vi "Dashboard Main.vi"() -> ()   [LabVIEW 2012]
uses:
  <vilib>/event_ctls.llb/eventvkey.ctl
  <vilib>/Utility/config.llb/Read Key (String).vi
  <vilib>/Utility/config.llb/Read Key (I32).vi
  <vilib>/Utility/config.llb/Write Key (String).vi
  <vilib>/Utility/config.llb/Write Key (I32).vi
  <vilib>/Utility/config.llb/NI_LVConfig.lvlib
panel:
  in  "Camera Settings":T1={"Frate Rate"=30, "Compression"=30, "Size"=1} {"Frate Rate" scale=1.0..30.0; "Size" items=["640x480", "320x240", "160x120"]}
  out "Mode":T2(ring)=enum."Auto Disabled"
  out "Camera IP":string
  in  "Dashboard Tab":T3(tab)
  in  "Reverse":bool
  in  "Control Mode":string(combo)="Tank: Dual Joystick"
  out "Lifting?":bool
  out "Lifting Enabled?":bool caption="Launching Enabled"
  out "Ready to fire?":bool
  out "Firing?":bool
  out "Launching Enabled?":bool caption="Launching Enabled"
  out "JS1 Z":dbl(slide) scale=-1.0..1.0 scale format="%#_2e"
  out "JS2 Z":dbl(slide) scale=-1.0..1.0 scale format="%#_2e"
  out "Joystick 1":cluster{"X":dbl, "Y":dbl}[](graph)
  out "Joystick 2":cluster{"X":dbl, "Y":dbl}[](graph)
  out "JS Buttons 1":T4
  out "JS Buttons 2":T4
  out "MotorSlide4":dbl(slide) scale=-1.0..1.0 scale format="%#_2e"
  out "MotorSlide3":dbl(slide) scale=-1.0..1.0 scale format="%#_2e"
  out "MotorSlide2":dbl(slide) scale=-1.0..1.0 scale format="%#_2e"
  in  "MotorName3":string="Front Left"
  in  "MotorName4":string="Front Right"
  in  "MotorName1":string="Rear Left"
  in  "MotorName2":string="Rear Right"
  out "MotorChart4":dbl(graph)
  out "MotorChart3":dbl(graph)
  out "MotorChart2":dbl(graph)
  out "MotorSlide1":dbl(slide) scale=-1.0..1.0 scale format="%#_2e"
  out "MotorChart1":dbl(graph)
  out "Battery Value":dbl(slide) scale=0.0..14.0 scale format="%#_2e"
  out "Battery":sgl(graph)
  out "Robot IP":string
  out "Motor Speed":dbl
  out "Throttle Speed":dbl
  in  "DB Camera Config":bool
  in  "Enable":bool=TRUE
  out "Mbps 2":dbl format="%#.1g"
  out "fps":dbl format="%#.1g"
  out "Mbps":bool
  in  "Slider":dbl(slide) scale=0.0..100.0 scale format="%#_3g"
  in  "On/Off":bool caption="Solenoid"
  in  "Test Name":u16(ring) items=["Select the test to run...", "Example Test", "-------------------------------", "List of tests is built in robot code.", "Replace with your own automated tests."]
  in  "Test Tree":string(tree)
  in  "Motor":cluster{"Value":dbl, "Enable":bool} {"Value" scale=-1.0..1.0 scale format="%#_3g"}
  out "Progress":T5 {"Test Progress" scale=0.0..100.0}
  in  "Rev/Fwd":cluster{"Forward":bool, "Reverse":bool}
  in  "Ring":u16(ring) items=["Auto", "Fixed indoor", "Fixed outdoor 1", "Fixed outdoor 2", "Fixed fluorescent 1", "Fixed fluorescent 2", "Hold current"]
  in  "Listbox":i32(listbox)
  in  "Viewer":T6(tab)
  out "Image Error Message":string="Timeout in Camera Communications"
  out "Camera Image":T7(plugin-control)
  out "Buttons 1":cluster{"1":bool, "2":bool, "3":bool}
  out "Kinect 1":cluster{"X":dbl, "Y":dbl, "Z":dbl} {"X" scale=1.0..-1.0; "Y" scale=1.0..-1.0; "Z" scale=1.0..-1.0}
  out "Buttons 2":cluster{"1":bool, "2":bool, "3":bool}
  out "Kinect 2":cluster{"X":dbl, "Y":dbl, "Z":dbl} {"X" scale=1.0..-1.0; "Y" scale=1.0..-1.0; "Z" scale=1.0..-1.0}
  out "Version":string
  out "Skeleton Picture":picture
  out "Players":i8
  out "Tree":string(tree)
  # "Robot IP:"
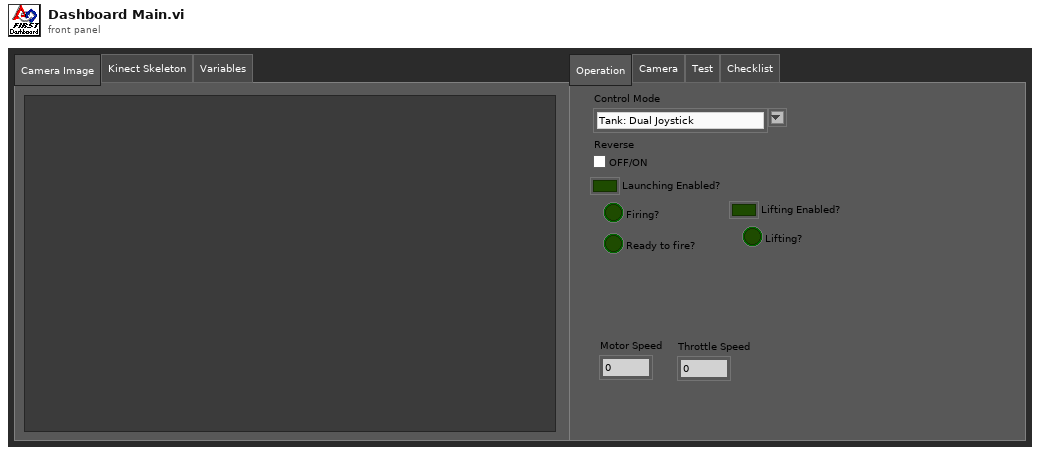
[diagram p1: front panel]
types:
  T1 = cluster{"Frate Rate":i32, "Compression":i32, "Size":u16}
  T2 = enum8{"Tele-Op Disabled", "Tele-Op Enabled", "Auto Disabled", "Auto Enabled", "Test Disabled", "Test Enabled", ""}
  T3 = enum32{"Operation", "Camera", "Test", "Checklist"}
  T4 = cluster{bool, bool, bool, bool, bool, bool, bool, bool, bool, bool, bool, bool}
  T5 = cluster{"Test Progress":u8, "Test Progress Text":string}
  T6 = enum32{"Camera Image", "Kinect Skeleton", "Variables"}
  T7 = typedef "IMAQ Image.ctl" = refnum<image>
  T8 = typedef "Image Type" = u32
  T9 = typedef "LVBoundsTypeDef.ctl" = cluster{"Width":u32, "Height":u32}
  T10 = typedef "SkeletonTrackState.ctl" = enum32{"NotTracked", "PositionOnly", "Tracked"}
  T11 = cluster{"TrackingState":u8[], "Position":cluster{"x":sgl, "y":sgl, "z":sgl}, cluster{"x":sgl, "y":sgl, "z":sgl, sgl}[], "TrackState":T10}
  T12 = cluster{cluster{"ScaledToPercentRange":dbl, "ScaledToPercentRange":dbl, "ScaledToPercentRange":dbl}, cluster{bool, bool, bool}}[]
  T13 = cluster{cluster{"ScaledToPercentRange":dbl, "ScaledToPercentRange":dbl, "ScaledToPercentRange":dbl}, cluster{bool, bool, bool}}
  T14 = cluster{"ScaledToPercentRange":dbl, "ScaledToPercentRange":dbl, "ScaledToPercentRange":dbl}
  T15 = typedef "LVRectTypeDef.ctl" = cluster{"Left":i16, "Top":i16, "Right":i16, "Bottom":i16}
  T16 = cluster{"Competition mode":bool, "Robot Link":bool, "Autonomous":bool, "Enabled":bool, "E-Stop":bool, "Simulated":bool, "TestMode":bool, "Docked Window":bool}
  T17 = cluster{"Boolean Array[0]":bool, "Boolean Array[1]":bool, "Boolean Array[2]":bool, "Boolean Array[3]":bool, "Boolean Array[4]":bool, "Boolean Array[5]":bool, "Boolean Array[6]":bool, "Boolean Array[7]":bool, "Boolean Array[8]":bool, "Boolean Array[9]":bool, "Boolean Array[10]":bool, "Boolean Array[11]":bool}
  T18 = typedef "NI_LVConfig.lvlib/Config Data RefNum.ctl" = refnum<k1>
  T19 = typedef "eventvkey.ctl" = enum16{"ASCII", "Enter", "Return", "Shift", "Ctrl", "Alt", "Cmd", "Opt", "Caps", "NumLock", "Clear", "Break", "Up", "Down", "Left", "Right", "Insert", "Delete", "Home", "End", "PageUp", "PageDown", "Escape", "Help", "Pause", "ScrollLock", "F1", "F2", "F3", "F4", "F5", "F6", "F7", "F8", "F9", "F10", "F11", "F12", "F13", "F14", "F15", "F16", "F17", "F18", "F19", "F20", "F21", "F22", "F23", "F24", "Play", "VolumeUp", "VolumeDown", "Mute", "Two Byte Char"}
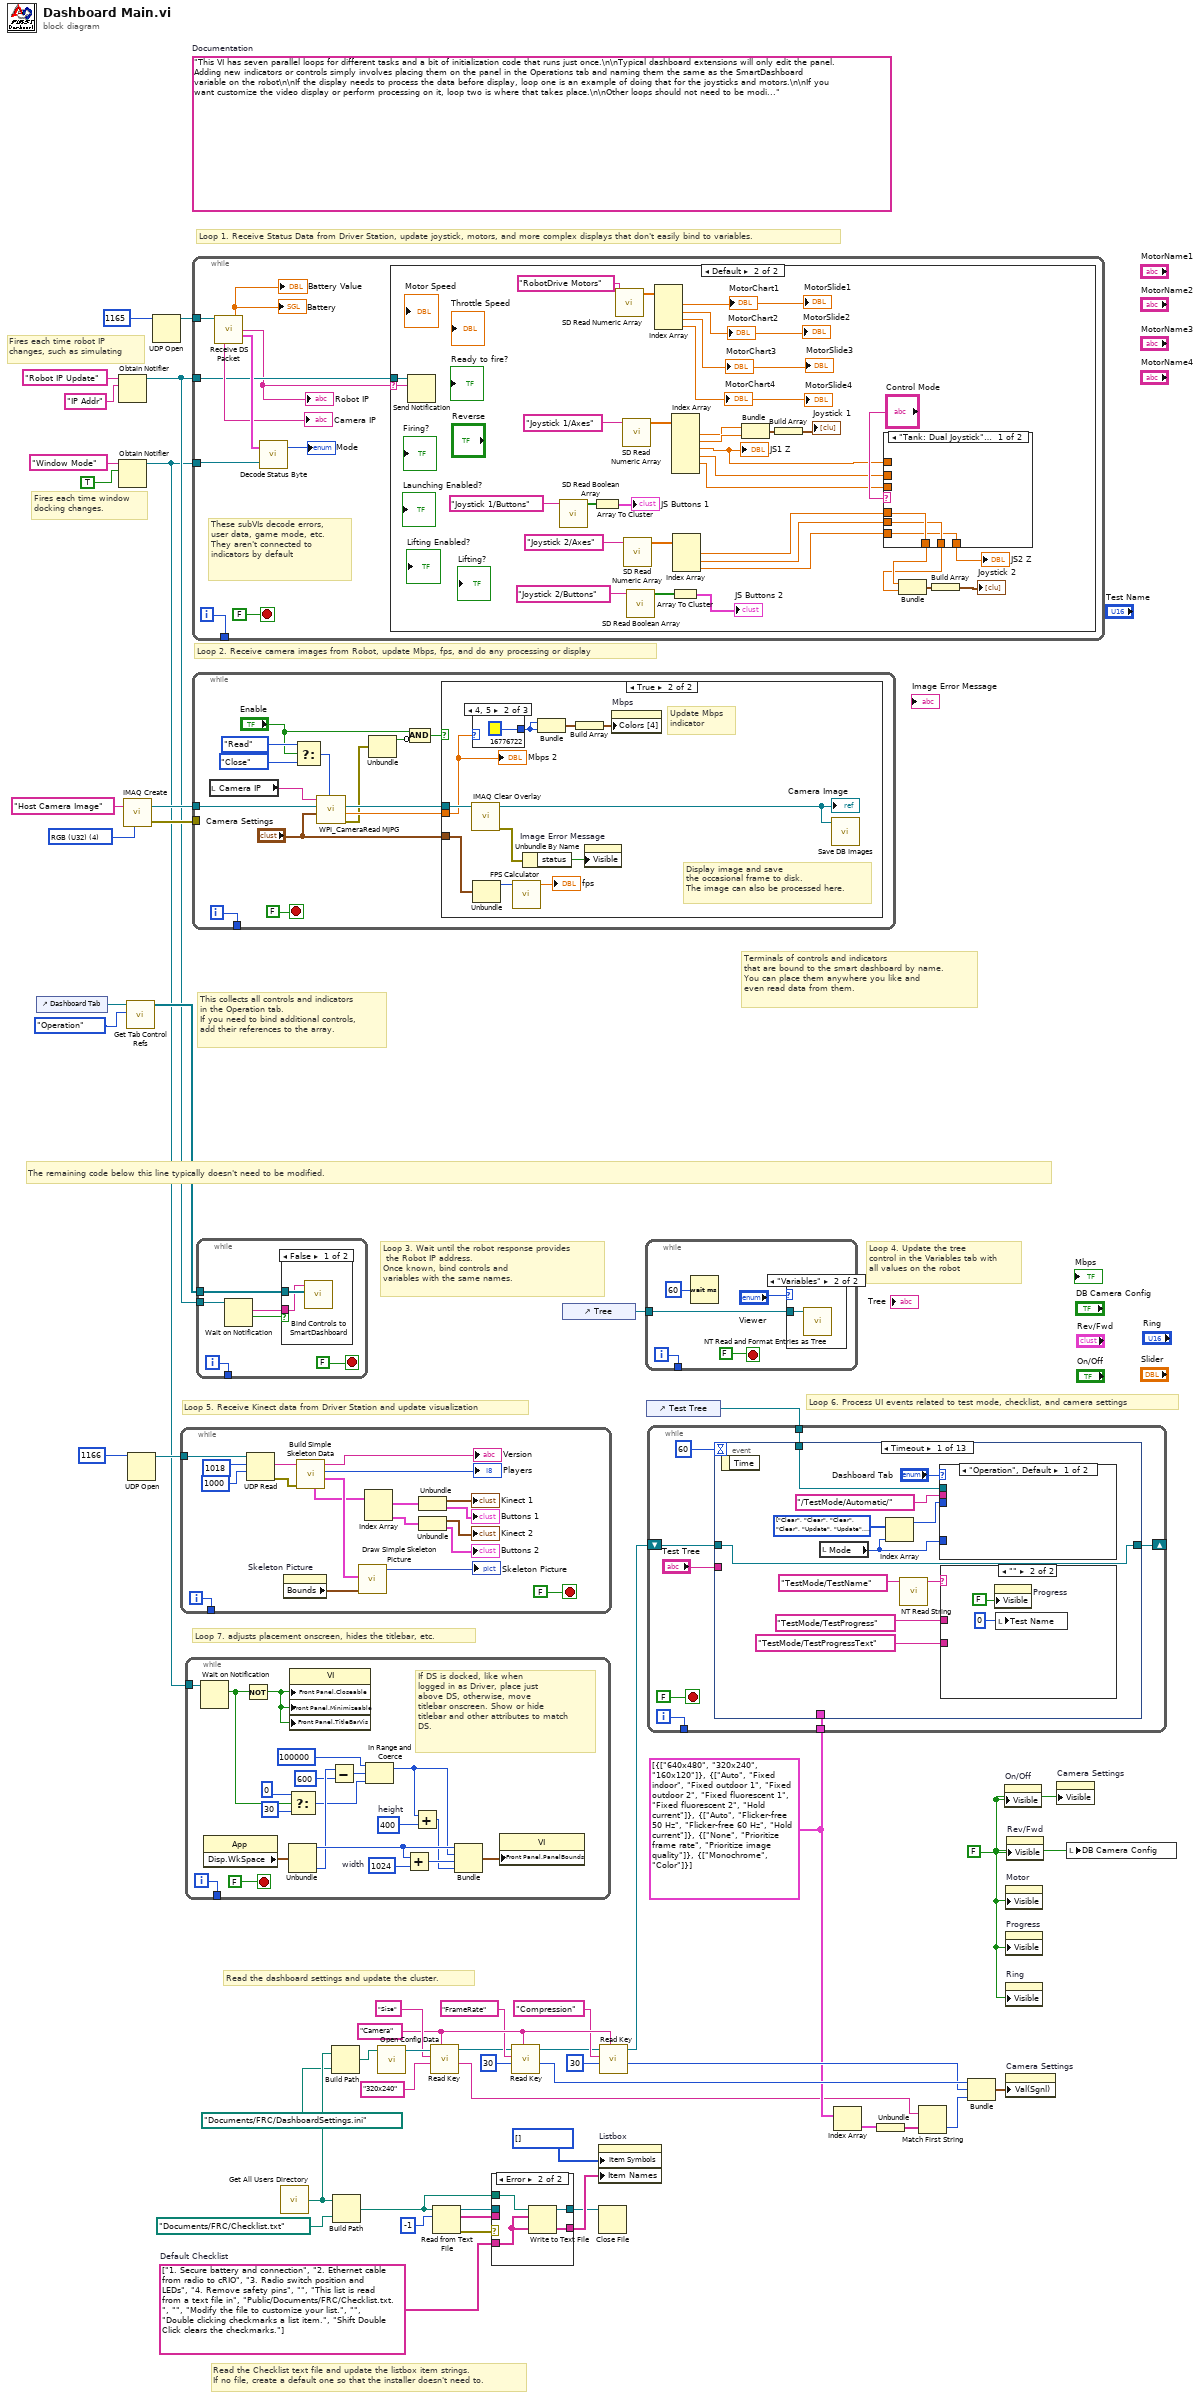
[diagram p0: block diagram]
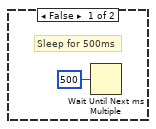
[diagram p3: hidden frame]
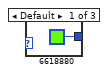
[diagram p4: hidden frame]
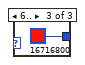
[diagram p5: hidden frame]
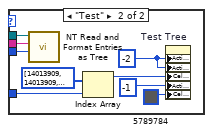
[diagram p7: hidden frame]
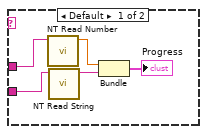
[diagram p8: hidden frame]
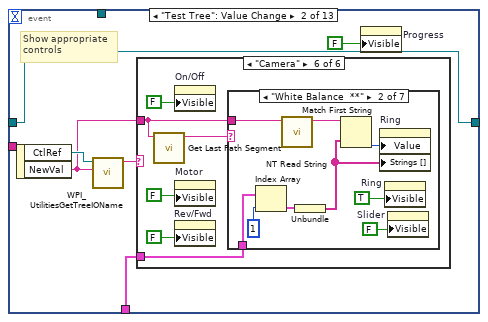
[diagram p9: hidden frame]
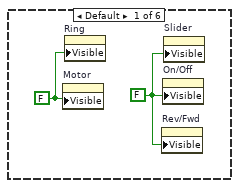
[diagram p10: hidden frame]
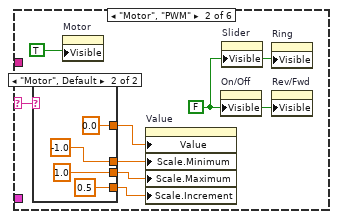
[diagram p11: hidden frame]
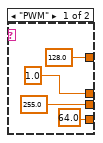
[diagram p12: hidden frame]
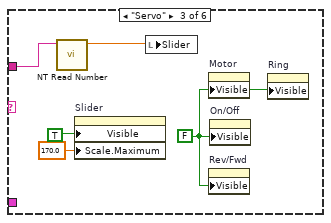
[diagram p13: hidden frame]
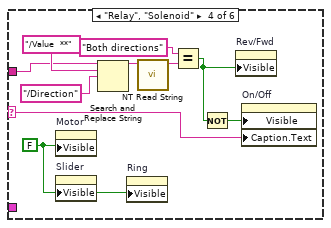
[diagram p14: hidden frame]
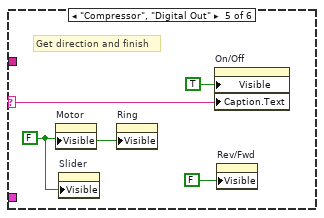
[diagram p15: hidden frame]
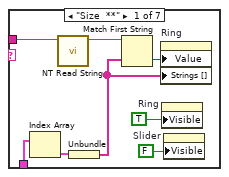
[diagram p16: hidden frame]
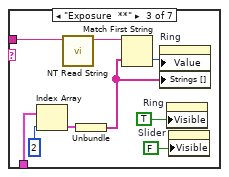
[diagram p17: hidden frame]
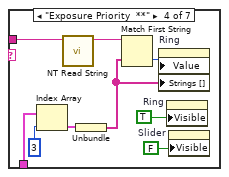
[diagram p18: hidden frame]
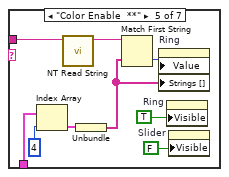
[diagram p19: hidden frame]
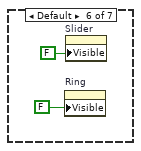
[diagram p20: hidden frame]
diagram:
  w21 = "Camera"
  w13 = cluster{string[]}[] [{["640x480", "320x240", "160x120"]}, {["Auto", "Fixed indoor", "Fixed outdoor 1", "Fixed outdoor 2", "Fixed fluorescent 1", "Fixed fluorescent 2", "Hold current"]}, {["Auto", "Flicker-free 50 Hz", "Flicker-free 60 Hz", "Hold current"]}, {["None", "Prioritize frame rate", "Prioritize image quality"]}, {["Monochrome", "Color"]}]
  w29 = string[] ["1. Secure battery and connection", "2. Ethernet cable from radio to cRIO", "3. Radio switch position and LEDs", "4. Remove safety pins", "", "This list is read from a text file in", "Public/Documents/FRC/Checklist.txt.", "", "Modify the file to customize your list.", "", "Double clicking checkmarks a list item.", "Shift Double Click clears the checkmarks."]  # Default Checklist
  w27 = FALSE ("Visible")
  (unwired) "This VI has seven parallel loops for different tasks and a bit of initialization code that runs just once.\n\nTypical dashboard extensions will only edit the panel. Adding new indicators or controls simply involves placing them on the panel in the Operations tab and naming them the same as the SmartDashboard variable on the robot\n\nIf the display needs to process the data before display, loop one is an example of doing that for the joysticks and motors.\n\nIf you want customize the video display or perform processing on it, loop two is where that takes place.\n\nOther loops should not need to be modified. They are pretty standard, and document the task they perform."  # Documentation
  w50 = T8 4 items=["Grayscale (U8)", "Grayscale (I16)", "Grayscale (SGL)", "Complex (CSG)", "RGB (U32)", "HSL (U32)", "RGB (U64)"] ("Image Type")
  # "Fires each time robot IP\nchanges, such as simulating"
  # "Fires each time window\ndocking changes."
  # "Read the Checklist text file and update the listbox item strings.\nIf no file, create a default one so that the installer doesn't need to."
  # "This collects all controls and indicators\nin the Operation tab.\nIf you need to bind additional controls,\nadd their references to the array."
  # "The remaining code below this line typically doesn't need to be modified."
  # "Loop 6. Process UI events related to test mode, checklist, and camera settings"
  # "Read the dashboard settings and update the cluster."
  # "Terminals of controls and indicators\nthat are bound to the smart dashboard by name.\nYou can place them anywhere you like and\neven read data from them."
  # "Loop 4. Update the tree\ncontrol in the Variables tab with\nall values on the robot"
  # "Loop 3. Wait until the robot response provides\n the Robot IP address.\nOnce known, bind controls and\nvariables with the same names."
  # "Loop 5. Receive Kinect data from Driver Station and update visualization"
  # "Loop 7. adjusts placement onscreen, hides the titlebar, etc."
  # "Loop 1. Receive Status Data from Driver Station, update joystick, motors, and more complex displays that don't easily bind to variables."
  # "Loop 2. Receive camera images from Robot, update Mbps, fps, and do any processing or display"
  n1 = control-ref of="Dashboard Tab"() -> (w43:refnum<vi>)
  n2 = Obtain Notifier(name (unnamed)="Robot IP Update", notification data type="IP Addr" ("name (unnamed)")) -> (notifier out=w40:refnum<notifier>)  [unwired: 2 in, 2 out]
  n3 = Obtain Notifier(name (unnamed)="Window Mode", notification data type=TRUE) -> (notifier out=w33:refnum<notifier>)  [unwired: 2 in, 2 out]
  n4 = call "IMAQ Create"("Image Name"="Host Camera Image", "Image Type"=w50) -> ("New Image"=w48:T7, "error out"=w47:errorcluster)  [unwired: 2 in, 1 out]
  n5 = call <vilib>:"Get Tab Control Refs.vi"("Page Index"=enum32{"Operation", "Test"}."Operation" ("Dashboard Tab"), "TabControl in"=w43) -> ("ControlsOnPage"=w44:refnum<vi>[])  [unwired: 9 in]
  n6 = UDP Open(11:u16 1166 ("port")) -> (port=w45:refnum<k16>)  [unwired: 2 in, 4 out]
  n7 = UDP Open(11:u16 1165 ("port")) -> (port=w51:refnum<k16>)  [unwired: 2 in, 4 out]
  n8 = while {
    tunnel: w45 -> [w69]
    tunnel: [w54] -> _
    i -> [w54]
    stop <- FALSE stop-if-true
    n9 = UDP Read(connection ID=w69, max size (548)=1018 ("bytes to read"), timeout ms (25000)=1000) -> (data out=w63:string, error out=w53:errorcluster)  [unwired: 1 in, 3 out]
    n10 = property on="Skeleton Picture" class="Pict"() -> ("Bounds"=w65:T9)  [unwired: 2 in, 2 out]
    n11 = call "Build Simple Skeleton Data.vi"("error in (no error)"=w53, "data in"=w63) -> ("Skeleton Data"=w64:T11, "NumPlayers"=→"Players":i8, "Version String"=→"Version":string, "Simple Joystick Info"=w61:T12)  [unwired: 5 in, 1 out]
    n12 = call "Draw Simple Skeleton Picture.vi"("Bounds"=w65, "Simple Skeleton"=w64) -> ("new picture out"=→"Skeleton Picture":picture)  [unwired: 9 in]
    n13 = Index Array(array=w61) -> (element #1=w60:T13, element #2=w59:T13)  [unwired: 2 in]
    n14 = Unbundle(w60) -> (→"Kinect 1":T14, →"Buttons 1":cluster{bool, bool, bool})
    n15 = Unbundle(w59) -> (→"Kinect 2":T14, →"Buttons 2":cluster{bool, bool, bool})
  }
  n16 = while {
    tunnel: w33 -> [w90]
    tunnel: [w88] -> _
    i -> [w88]
    stop <- FALSE stop-if-true
    w80 = 1024  # width
    w83 = 400  # height
    # "If DS is docked, like when\nlogged in as Driver, place just\nabove DS, otherwise, move\ntitlebar onscreen. Show or hide\ntitlebar and other attributes to match\nDS."
    n17 = Wait on Notification(notifier=w90) -> (notification=w75:bool)  [unwired: 3 in, 3 out]
    n18 = property class="App"() -> ("Disp.WkSpace"=w86:T15)  [unwired: 2 in, 2 out]
    n19 = Not(x=w75) -> (.not. x?=w89:bool)
    n20 = Unbundle(w86) -> ("Left"=w84:i16, "Bottom"=w81:i16)  [unwired: 2 out]
    n21 = Select(t=0, s=w75, f=30) -> (s? t:f=w74:i32)
    n22 = property class="VI"("Front Panel.Closeable"=w89, "Front Panel.Minimizeable"=w89, "Front Panel.TitleBarVis"=w89) -> ()  [unwired: 2 in, 2 out]
    n23 = Subtract(x=w81, y=600) -> (x-y=w78:i32)
    n24 = In Range and Coerce(upper limit=100000, x=w78, lower limit=w74) -> (coerced(x)=w72:i32)  [unwired: 1 out]
    n25 = Add(x=w84, y=w80) -> (x+y=w85:i32)
    n26 = Add(x=w72, y=w83) -> (x+y=w82:i32)
    n27 = Bundle("Left"=w84, w72, w85, w82) -> (w87:cluster{"Left":i16, i32, i32, i32})  [unwired: 1 out]
    n28 = property class="VI"("Front Panel.PanelBounds"=w87) -> ()  [unwired: 2 in, 2 out]
  }
  n29 = while {
    tunnel: w48 -> [w101]
    tunnel: w47 -> [_]
    tunnel: [w104] -> _
    i -> [w104]
    stop <- FALSE stop-if-true
    n30 = local read "Camera IP"() -> (w103:string)
    n31 = Select(t=enum16{"Read", "Reopen", "Close"}."Read" ("Operation"), s="Enable", f=enum16{"Read", "Reopen", "Close"}."Close" ("Operation")) -> (s? t:f=w96:enum16{"Read", "Reopen", "Close"})
    n32 = call <vilib>:"WPI_CameraRead MJPG.vi"("Operation"=w96, "Camera Settings"="Camera Settings", "Image"=w101, "address"=w103) -> ("error out"=w95:errorcluster, "Bandwidth (kbps)"=w99:dbl, "Image Out"=w100:T7)  [unwired: 5 in]
    n33 = Unbundle(w95) -> ("status"=w93:bool)  [unwired: 2 out]
    n34 = Compound Arithmetic op=AND("Enable", invert w93) -> (w92:bool)
    n35 = case shown="True" w92 {
      tunnel: "Camera Settings" -> [_ w108]
      tunnel: w100 -> [_ w111]
      tunnel: w99 -> [_ w110]
      frame False {
        # "Sleep for 500ms"
        n36 = Wait Until Next ms Multiple(millisecond multiple=u32 500) -> ()  [unwired: 1 out]
      }
      frame True {
        # "Display image and save\nthe occasional frame to disk.\nThe image can also be processed here."
        # "Update Mbps\nindicator"
        n37 = call "IMAQ Clear Overlay"("Image"=w111) -> ("error out"=w116:errorcluster, "Image Out"=w115:T7)  [unwired: 2 in, 7 out]
        "Camera Image" <- w115
        n38 = case shown="4, 5" w110 {
          tunnel: [u32 6618880 ("Color Box") u32 16776722 ("Color Box") u32 16716800 ("Color Box")] -> w112
          frame Default {
          }
          frame 4, 5 {
          }
          frame 6.. {
          }
        }
        n39 = Unbundle(w108) -> ("Frate Rate"=w107:i32)  [unwired: 2 out]
        n40 = call "FPS Calculator.vi"("Average Count"=w107) -> ("fps"=→"fps":dbl)  [unwired: 10 in]
        n41 = Unbundle By Name(w116) -> ("status"=w117:bool)
        n42 = Bundle("Color Box"=w112, "Color Box"=w112) -> (w114:cluster{"Color Box":u32, "Color Box":u32})  [unwired: 1 out]
        n43 = Build Array(w114) -> (w113:cluster{"Color Box":u32, "Color Box":u32}[])
        n44 = property on="Image Error Message" class="Str"("Visible"=w117) -> ()  [unwired: 2 in, 2 out]
        n45 = property on="Mbps" class="Bool (strict)"("Colors [4]"=w113) -> ()  [unwired: 2 in, 2 out]
        n46 = call "Save DB Images.vi"("Image"=w115) -> ()  [unwired: 2 in, 1 out]
        "Mbps 2" <- w110
      }
    }
  }
  n47 = while {
    tunnel: w51 -> [w128]
    tunnel: w40 -> [w122]
    tunnel: w33 -> [w126]
    tunnel: [w123] -> _
    i -> [w123]
    stop <- FALSE stop-if-true
    # "These subVIs decode errors, user data, game mode, etc.\nThey aren't connected to indicators by default"
    n48 = call "Receive DS Packet.vi"("Recv Socket"=w128) -> ("Battery"=→"Battery" →"Battery Value":sgl, "Robot IP Address"=w121:string, "Status"=w129:T16, "Camera IP Address"=→"Camera IP":string)  [unwired: 1 in, 10 out]
    "Robot IP" <- w121
    n49 = call "Decode Status Byte.vi"("Window Mode Notifier"=w126, "Status"=w129) -> ("Mode"=→"Mode":T2)  [unwired: 1 out]
    n50 = case shown="Default" w121 {
      selector: w121 -> [_ w142]
      tunnel: w122 -> [_ w143]
      frame "0.0.0.0" {
        # "Robot not responding, don't poll the variables"
      }
      frame Default {
        n51 = Send Notification(notification=w142, notifier=w143) -> ()  [unwired: 1 in, 2 out]
        n52 = call <vilib>:"SD Read Boolean Array.vi"("Name"="Joystick 1/Buttons") -> ("Boolean Array"=w156:bool[])  [unwired: 8 in, 2 out]
        n53 = Array To Cluster(array=w156) -> (cluster=→"JS Buttons 1":T17)
        n54 = call <vilib>:"SD Read Numeric Array.vi"("Name"="RobotDrive Motors") -> ("Numeric Array"=w161:dbl[])  [unwired: 8 in, 2 out]
        n55 = call <vilib>:"SD Read Numeric Array.vi"("Name"="Joystick 1/Axes") -> ("Numeric Array"=w154:dbl[])  [unwired: 8 in, 2 out]
        n56 = call <vilib>:"SD Read Numeric Array.vi"("Name"="Joystick 2/Axes") -> ("Numeric Array"=w149:dbl[])  [unwired: 8 in, 2 out]
        n57 = call <vilib>:"SD Read Boolean Array.vi"("Name"="Joystick 2/Buttons") -> ("Boolean Array"=w148:bool[])  [unwired: 8 in, 2 out]
        n58 = Index Array(array=w161) -> (element #1=→"MotorChart1" →"MotorSlide1":dbl, element #2=→"MotorSlide2" →"MotorChart2":dbl, element #3=→"MotorChart3" →"MotorSlide3":dbl, element #4=→"MotorChart4" →"MotorSlide4":dbl)  [unwired: 4 in]
        n59 = Index Array(array=w154) -> (element #1=w152:dbl, element #2=w153:dbl, element #3=w138:dbl, element #4=w139:dbl, element #5=w140:dbl)  [unwired: 6 in, 1 out]
        "JS1 Z" <- w138
        n60 = Array To Cluster(array=w148) -> (cluster=→"JS Buttons 2":T17)
        n61 = Index Array(array=w149) -> (element #1=w137:dbl, element #2=w136:dbl, element #3=w135:dbl)  [unwired: 3 in]
        n62 = Bundle("Numeric"=w152, "Numeric"=w153) -> (w151:cluster{"Numeric":dbl, "Numeric":dbl})  [unwired: 1 in]
        n63 = Build Array(w151) -> (→"Joystick 1":cluster{"Numeric":dbl, "Numeric":dbl}[])
        n64 = case shown="\"Tank: Dual Joystick\", Default" "Control Mode" {
          tunnel: w140 -> [_ w169]
          tunnel: w139 -> [_ w170]
          tunnel: w138 -> [_ w168]
          tunnel: w137 -> [w167 _]
          tunnel: w136 -> [w166 _]
          tunnel: w135 -> [w165 _]
          tunnel: [w167 w170] -> w134
          tunnel: [w166 w169] -> w133
          tunnel: [w165 w168] -> w132
          frame "Tank: Dual Joystick", Default {
          }
          frame "Tank: 360 Gamepad" {
          }
        }
        "JS2 Z" <- w132
        n65 = Bundle("Numeric"=w134, "Numeric"=w133) -> (w145:cluster{"Numeric":dbl, "Numeric":dbl})  [unwired: 1 in]
        n66 = Build Array(w145) -> (→"Joystick 2":cluster{"Numeric":dbl, "Numeric":dbl}[])
      }
    }
  }
  n67 = while {
    tunnel: w44 -> [w176]
    tunnel: w40 -> [w173]
    tunnel: [w171] -> _
    i -> [w171]
    stop <- FALSE stop-if-true
    n68 = Wait on Notification(notifier=w173) -> (notification=w172:string, timed out?=w174:bool)  [unwired: 3 in, 2 out]
    n69 = case shown="False" w174 {
      tunnel: w176 -> [w178 _]
      tunnel: w172 -> [w177 _]
      frame False {
        n70 = call <vilib>:"Bind Controls to SmartDashboard.vi"("Bound Control Refs"=w178, "Server IP Address"=w177) -> ()  [unwired: 10 in]
      }
      frame True {
      }
    }
  }
  n71 = call "Get All Users Directory.vi"() -> ("All User Path"=w26:path)
  n72 = Build Path(base path=w26, name or relative path=path "Documents/FRC/DashboardSettings.ini") -> (appended path=w25:path)
  n73 = Build Path(base path=w26, name or relative path=path "Documents/FRC/Checklist.txt") -> (appended path=w30:path)
  n74 = call <vilib>:"Open Config Data.vi"("configuration file path"=w25) -> ("refnum"=w24:T18)  [unwired: 8 in, 2 out]
  n75 = call-poly <vilib>:"Read Key.vi"("section"=w21, "default value"="320x240", "key"="Size", "refnum"=w24) -> ("value"=w11:string, "refnum out"=w6:T18)  [unwired: 2 in, 4 out]
  n76 = Read from Text File(file (use dialog)=w30, count=-1 ("timeout ms (25000)")) -> (refnum out=w8:refnum<file>, text=w31:string[], error out=w32:errorcluster)  [unwired: 2 in, 1 out]
  n77 = case shown="Error" w32 {
    tunnel: w31 -> [w180 _]
    tunnel: [w180 w182] -> w28
    tunnel: w29 -> [_ w182]
    tunnel: w30 -> [_ w183]
    tunnel: [w179 w181] -> w7
    tunnel: w8 -> [w179 _]
    frame No Error {
    }
    frame Error {
      n78 = Write to Text File(file (use dialog)=w183, text=w182) -> (refnum out=w181:refnum<file>)  [unwired: 2 in, 2 out]
    }
  }
  n79 = call-poly <vilib>:"Read Key.vi"("section"=w21, "default value"=30, "key"="FrameRate", "refnum"=w6) -> ("value"=w16:i32, "refnum out"=w5:T18)  [unwired: 1 in, 5 out]
  n80 = control-ref of="Tree"() -> (w2:refnum<vi>)
  n81 = property on="Listbox" class="LstBox (strict)"("Item Symbols"=i32[] [], "Item Names"=w28) -> ()  [unwired: 2 in, 2 out]
  n82 = Close File(refnum=w7) -> ()  [unwired: 1 in, 2 out]
  n83 = call-poly <vilib>:"Read Key.vi"("section"=w21, "default value"=30, "key"="Compression", "refnum"=w5) -> ("value"=w15:i32, "refnum out"=w3:T18)  [unwired: 1 in, 5 out]
  n84 = while {
    tunnel: [w185] -> _
    tunnel: w2 -> [w184]
    i -> [w185]
    stop <- FALSE stop-if-true
    n85 = Wait (ms)(milliseconds to wait=u32 60) -> ()  [unwired: 1 out]
    n86 = case shown="\"Variables\"" "Viewer" {
      tunnel: w184 -> [_ w189]
      frame Default {
      }
      frame "Variables" {
        n87 = call <vilib>:"NT Read and Format Entries as Tree.vi"("Tree Refnum"=w189) -> ()  [unwired: 9 in, 2 out]
      }
    }
  }
  n88 = control-ref of="Test Tree"() -> (w1:refnum<vi>)
  n89 = while {
    tunnel: w13 -> [w194]
    shift-right: [w193] -> _
    shift-left: w3 -> [w192]
    tunnel: [w191] -> _
    tunnel: w1 -> [w190]
    i -> [w191]
    stop <- FALSE stop-if-true
    n90 = event shown="[0] Timeout" {
      selector: _ -> [_ _ _ _ _ _ _ _ _ _ _ _ _]
      dyn-events: _ -> [_ _ _ _ _ _ _ _ _ _ _ _ _]
      timeout: u32 60 ("milliseconds to wait") -> [_ _ _ _ _ _ _ _ _ _ _ _ _]
      tunnel: w190 -> [w204 _ _ _ _ _ _ _ _ _ _ _ _]
      tunnel: "Test Tree" -> [_ _ _ _ _ _ _ _ w398 w406 w408 w412 w420]
      tunnel: w194 -> [_ w226 _ _ _ _ w362 w392 _ _ _ _ _]
      tunnel: [w198 w225 _ w328 w336 w348 w361 w385 w397 w404 w407 w411 w419] -> w193
      tunnel: w192 -> [w198 w225 _ w328 w336 w348 w360 w385 w397 w404 w407 w411 w419]
      event Timeout {
        w203 = enum16{"Update", "Clear"}[] [enum."Clear", enum."Clear", enum."Clear", enum."Clear", enum."Update", enum."Update", enum."Clear"] items=["Update", "Clear"]
        n91 = event-data() -> ()  [unwired: 1 in, 1 out]
        n92 = local read "Mode"() -> (w201:T2)
        n93 = Index Array(array=w203, index=w201) -> (element=w202:enum16{"Update", "Clear"})
        n94 = call <vilib>:"NT Read String.vi"("Name"="TestMode/TestName") -> ("String"=w207:string)  [unwired: 9 in, 1 out]
        n95 = case shown="\"Operation\", Default" "Dashboard Tab" {
          tunnel: w204 -> [_ w217]
          tunnel: "/TestMode/Automatic/" ("Name Pattern") -> [_ w216]
          tunnel: w202 -> [_ w215]
          tunnel: w201 -> [_ w213]
          frame "Operation", Default {
          }
          frame "Test" {
            w212 = -2 ("Active Item:Row Number")
            n96 = call <vilib>:"NT Read and Format Entries as Tree.vi"("Operation"=w215, "Name Pattern"=w216, "Tree Refnum"=w217) -> ()  [unwired: 7 in, 2 out]
            n97 = Index Array(array=u32[] [14013909, 14013909, 14013909, 14013909, 14013909, 16777215, 14013909], index=w213) -> (element=w211:u32)
            n98 = property on="Test Tree" class="Tree (strict)"("Active Item Row Number"=w212, "ActiveColNum"=w212, "CellBG"=w211, "Active Item Row Number"=-1 ("Active Item:Row Number"), "CellBG"=u32 5789784 ("Color Box")) -> ()  [unwired: 2 in, 2 out]
          }
        }
        n99 = case shown="\"\"" w207 {
          tunnel: "TestMode/TestProgress" ("Name") -> [w219 _]
          tunnel: "TestMode/TestProgressText" ("Name") -> [w218 _]
          frame Default {
            n100 = call <vilib>:"NT Read Number.vi"("Name"=w219) -> ("Numeric"=w220:dbl)  [unwired: 9 in, 1 out]
            n101 = call <vilib>:"NT Read String.vi"("Name"=w218) -> ("String"=w221:string)  [unwired: 9 in, 1 out]
            n102 = Bundle("Numeric"=w220, "String"=w221) -> (→"Progress":cluster{"Numeric":dbl, "String":string})  [unwired: 1 in]
          }
          frame "" {
            n103 = property on="Progress" class="Clust (strict)"("Visible"=FALSE) -> ()  [unwired: 2 in, 2 out]
            n104 = local write "Test Name"(u16 0) -> ()
          }
        }
      }
      event "Test Tree": Value Change {
        # "Show appropriate\ncontrols"
        n105 = event-data() -> ("CtlRef"=w229:refnum<vi>, "NewVal"=w227:string)  [unwired: 1 in]
        n106 = call <vilib>:"WPI_UtilitiesGetTreeIOName.vi"("NewVal"=w227, "TreeControl in"=w229) -> ("I/O Name"=w230:string)  [unwired: 9 in]
        n107 = case shown="\"Camera\"" w230 {
          selector: w230 -> [_ w237 _ w255 w264 _]
          tunnel: w227 -> [_ _ w252 w254 _ w271]
          tunnel: w226 -> [_ _ _ _ _ w270]
          frame Default {
            w232 = FALSE ("Visible")
            w231 = FALSE ("Visible")
            n108 = property on="Motor" class="Clust (strict)"("Visible"=w231) -> ()  [unwired: 2 in, 2 out]
            n109 = property on="Ring" class="Ring (strict)"("Visible"=w231) -> ()  [unwired: 2 in, 2 out]
            n110 = property on="Rev/Fwd" class="Clust (strict)"("Visible"=w232) -> ()  [unwired: 2 in, 2 out]
            n111 = property on="On/Off" class="Bool (strict)"("Visible"=w232) -> ()  [unwired: 2 in, 2 out]
            n112 = property on="Slider" class="Slide (strict)"("Visible"=w232) -> ()  [unwired: 2 in, 2 out]
          }
          frame "Motor", "PWM" {
            w238 = FALSE ("Visible")
            n113 = case shown="\"Motor\", Default" w237 {
              tunnel: [1.0 ("Value") -1.0 ("Value")] -> w236
              tunnel: [255.0 ("Value") 1.0 ("Value")] -> w235
              tunnel: [128.0 ("Value") 0.0 ("Value")] -> w234
              tunnel: [64.0 ("Value") 0.5 ("Value")] -> w233
              frame "PWM" {
              }
              frame "Motor", Default {
              }
            }
            n114 = property on="Motor" class="Clust (strict)"("Visible"=TRUE) -> ()  [unwired: 2 in, 2 out]
            n115 = property on="Value" class="Slide (strict)"("Value"=w234, "Scale.Minimum"=w236, "Scale.Maximum"=w235, "Scale.Increment"=w233) -> ()  [unwired: 2 in, 2 out]
            n116 = property on="On/Off" class="Bool (strict)"("Visible"=w238) -> ()  [unwired: 2 in, 2 out]
            n117 = property on="Slider" class="Slide (strict)"("Visible"=w238) -> ()  [unwired: 2 in, 2 out]
            n118 = property on="Ring" class="Ring (strict)"("Visible"=w238) -> ()  [unwired: 2 in, 2 out]
            n119 = property on="Rev/Fwd" class="Clust (strict)"("Visible"=w238) -> ()  [unwired: 2 in, 2 out]
          }
          frame "Servo" {
            w250 = FALSE ("Visible")
            n120 = call <vilib>:"NT Read Number.vi"("Name"=w252) -> ("Numeric"=w251:dbl)  [unwired: 9 in, 1 out]
            n121 = property on="Slider" class="Slide (strict)"("Visible"=TRUE, "Scale.Maximum"=170.0 ("Scale.Range:Maximum")) -> ()  [unwired: 2 in, 2 out]
            n122 = local write "Slider"(w251) -> ()
            n123 = property on="Motor" class="Clust (strict)"("Visible"=w250) -> ()  [unwired: 2 in, 2 out]
            n124 = property on="Rev/Fwd" class="Clust (strict)"("Visible"=w250) -> ()  [unwired: 2 in, 2 out]
            n125 = property on="On/Off" class="Bool (strict)"("Visible"=w250) -> ()  [unwired: 2 in, 2 out]
            n126 = property on="Ring" class="Ring (strict)"("Visible"=w250) -> ()  [unwired: 2 in, 2 out]
          }
          frame "Relay", "Solenoid" {
            w253 = FALSE ("Visible")
            n127 = property on="Motor" class="Clust (strict)"("Visible"=w253) -> ()  [unwired: 2 in, 2 out]
            n128 = property on="Slider" class="Slide (strict)"("Visible"=w253) -> ()  [unwired: 2 in, 2 out]
            n129 = Search and Replace String(input string=w254, search string="/Value  **", replace string="/Direction") -> (result string=w260:string)  [unwired: 5 in, 3 out]
            n130 = property on="Ring" class="Ring (strict)"("Visible"=w253) -> ()  [unwired: 2 in, 2 out]
            n131 = call <vilib>:"NT Read String.vi"("Name"=w260) -> ("String"=w258:string)  [unwired: 9 in, 1 out]
            n132 = Equal?(x="Both directions", y=w258) -> (x = y?=w256:bool)
            n133 = Not(x=w256) -> (.not. x?=w257:bool)
            n134 = property on="Rev/Fwd" class="Clust (strict)"("Visible"=w256) -> ()  [unwired: 2 in, 2 out]
            n135 = property on="On/Off" class="Bool (strict)"("Visible"=w257, "Caption.Text"=w255) -> ()  [unwired: 2 in, 2 out]
          }
          frame "Compressor", "Digital Out" {
            w263 = FALSE ("Visible")
            # "Get direction and finish"
            n136 = property on="Motor" class="Clust (strict)"("Visible"=w263) -> ()  [unwired: 2 in, 2 out]
            n137 = property on="Slider" class="Slide (strict)"("Visible"=w263) -> ()  [unwired: 2 in, 2 out]
            n138 = property on="Ring" class="Ring (strict)"("Visible"=w263) -> ()  [unwired: 2 in, 2 out]
            n139 = property on="On/Off" class="Bool (strict)"("Visible"=TRUE, "Caption.Text"=w264) -> ()  [unwired: 2 in, 2 out]
            n140 = property on="Rev/Fwd" class="Clust (strict)"("Visible"=FALSE) -> ()  [unwired: 2 in, 2 out]
          }
          frame "Camera" {
            n141 = call <vilib>:"Get Last Path Segment.vi"("String in"=w271) -> ("String out"=w272:string)  [unwired: 10 in]
            n142 = property on="On/Off" class="Bool (strict)"("Visible"=FALSE) -> ()  [unwired: 2 in, 2 out]
            n143 = property on="Motor" class="Clust (strict)"("Visible"=FALSE) -> ()  [unwired: 2 in, 2 out]
            n144 = property on="Rev/Fwd" class="Clust (strict)"("Visible"=FALSE) -> ()  [unwired: 2 in, 2 out]
            n145 = case shown="\"White Balance  **\"" w272 {
              tunnel: w271 -> [w278 w287 w296 w305 w314 _ w320]
              tunnel: w270 -> [w276 w284 w293 w302 w311 _ _]
              frame "Size  **" {
                n146 = Index Array(array=w276) -> (element=w275:cluster{string[]})  [unwired: 1 in]
                n147 = call <vilib>:"NT Read String.vi"("Name"=w278) -> ("String"=w277:string)  [unwired: 9 in, 1 out]
                n148 = Unbundle(w275) -> (w273:string[])
                n149 = Match First String(2:w273, 3:w277) -> (0:w274:i32)  [unwired: 1 out]
                n150 = property on="Ring" class="Ring (strict)"("Value"=w274, "Strings []"=w273) -> ()  [unwired: 2 in, 2 out]
                n151 = property on="Ring" class="Ring (strict)"("Visible"=TRUE) -> ()  [unwired: 2 in, 2 out]
                n152 = property on="Slider" class="Slide (strict)"("Visible"=FALSE) -> ()  [unwired: 2 in, 2 out]
              }
              frame "White Balance  **" {
                n153 = Index Array(array=w284, index=1) -> (element=w285:cluster{string[]})
                n154 = call <vilib>:"NT Read String.vi"("Name"=w287) -> ("String"=w286:string)  [unwired: 9 in, 1 out]
                n155 = Unbundle(w285) -> (w282:string[])
                n156 = Match First String(2:w282, 3:w286) -> (0:w281:i32)  [unwired: 1 out]
                n157 = property on="Ring" class="Ring (strict)"("Value"=w281, "Strings []"=w282) -> ()  [unwired: 2 in, 2 out]
                n158 = property on="Ring" class="Ring (strict)"("Visible"=TRUE) -> ()  [unwired: 2 in, 2 out]
                n159 = property on="Slider" class="Slide (strict)"("Visible"=FALSE) -> ()  [unwired: 2 in, 2 out]
              }
              frame "Exposure  **" {
                n160 = Index Array(array=w293, index=2) -> (element=w294:cluster{string[]})
                n161 = call <vilib>:"NT Read String.vi"("Name"=w296) -> ("String"=w295:string)  [unwired: 9 in, 1 out]
                n162 = Unbundle(w294) -> (w290:string[])
                n163 = Match First String(2:w290, 3:w295) -> (0:w291:i32)  [unwired: 1 out]
                n164 = property on="Ring" class="Ring (strict)"("Value"=w291, "Strings []"=w290) -> ()  [unwired: 2 in, 2 out]
                n165 = property on="Ring" class="Ring (strict)"("Visible"=TRUE) -> ()  [unwired: 2 in, 2 out]
                n166 = property on="Slider" class="Slide (strict)"("Visible"=FALSE) -> ()  [unwired: 2 in, 2 out]
              }
              frame "Exposure Priority  **" {
                n167 = Index Array(array=w302, index=3) -> (element=w303:cluster{string[]})
                n168 = call <vilib>:"NT Read String.vi"("Name"=w305) -> ("String"=w304:string)  [unwired: 9 in, 1 out]
                n169 = Unbundle(w303) -> (w299:string[])
                n170 = Match First String(2:w299, 3:w304) -> (0:w300:i32)  [unwired: 1 out]
                n171 = property on="Ring" class="Ring (strict)"("Value"=w300, "Strings []"=w299) -> ()  [unwired: 2 in, 2 out]
                n172 = property on="Ring" class="Ring (strict)"("Visible"=TRUE) -> ()  [unwired: 2 in, 2 out]
                n173 = property on="Slider" class="Slide (strict)"("Visible"=FALSE) -> ()  [unwired: 2 in, 2 out]
              }
              frame "Color Enable  **" {
                n174 = Index Array(array=w311, index=4) -> (element=w312:cluster{string[]})
                n175 = call <vilib>:"NT Read String.vi"("Name"=w314) -> ("String"=w313:string)  [unwired: 9 in, 1 out]
                n176 = Unbundle(w312) -> (w308:string[])
                n177 = Match First String(2:w308, 3:w313) -> (0:w309:i32)  [unwired: 1 out]
                n178 = property on="Ring" class="Ring (strict)"("Value"=w309, "Strings []"=w308) -> ()  [unwired: 2 in, 2 out]
                n179 = property on="Ring" class="Ring (strict)"("Visible"=TRUE) -> ()  [unwired: 2 in, 2 out]
                n180 = property on="Slider" class="Slide (strict)"("Visible"=FALSE) -> ()  [unwired: 2 in, 2 out]
              }
              frame Default {
                n181 = property on="Ring" class="Ring (strict)"("Visible"=FALSE) -> ()  [unwired: 2 in, 2 out]
                n182 = property on="Slider" class="Slide (strict)"("Visible"=FALSE) -> ()  [unwired: 2 in, 2 out]
              }
              frame "Brightness  **", "Color Level  **", "Compression  **", "FPS  **", "Sharpness  **" {
                n183 = call <vilib>:"NT Read Number.vi"("Name"=w320) -> ("Numeric"=w319:dbl)  [unwired: 9 in, 1 out]
                n184 = local write "Slider"(w319) -> ()
                n185 = property on="Slider" class="Slide (strict)"("Visible"=TRUE, "Scale.Maximum"=100.0 ("Scale.Range:Maximum")) -> ()  [unwired: 2 in, 2 out]
                n186 = property on="Ring" class="Ring (strict)"("Visible"=FALSE) -> ()  [unwired: 2 in, 2 out]
              }
            }
          }
        }
        n187 = property on="Progress" class="Clust (strict)"("Visible"=FALSE) -> ()  [unwired: 2 in, 2 out]
      }
      event "Test Name": Mouse Enter {
        # "Populate the ring with the list of tests"
        n188 = event-data() -> ()  [unwired: 1 in, 1 out]
        n189 = call <vilib>:"NT Read String Array.vi"("Name"="TestMode/TestList") -> ("String Array"=w327:string[])  [unwired: 9 in, 1 out]
        n190 = Build Array (concatenate)("Select the test to run...", w327) -> (w326:string[])
        n191 = property on="Test Name" class="Ring (strict)"("Strings []"=w326) -> ()  [unwired: 2 in, 2 out]
      }
      event "Test Name": Value Change {
        w329 = FALSE ("Visible")
        # "Tell the robot the test name to run"
        n192 = event-data() -> ("NewVal"=w333:u16)  [unwired: 1 in]
        n193 = property on="Test Name" class="Ring (strict)"() -> ("Strings []"=w334:string[])  [unwired: 2 in, 2 out]
        n194 = local write "Progress"(T5 {"Test Progress"=0, "Test Progress Text"=""} ("Progress")) -> ()
        n195 = Index Array(array=w334, index=w333) -> (element=w332:string)
        n196 = call <vilib>:"NT Write String.vi"("String"=w332, "Name"="TestMode/TestName") -> ()  [unwired: 9 in, 1 out]
        n197 = property on="Progress" class="Clust (strict)"("Visible"=TRUE) -> ()  [unwired: 2 in, 2 out]
        n198 = property on="Motor" class="Clust (strict)"("Visible"=w329) -> ()  [unwired: 2 in, 2 out]
        n199 = property on="Slider" class="Slide (strict)"("Visible"=w329) -> ()  [unwired: 2 in, 2 out]
        n200 = property on="On/Off" class="Bool (strict)"("Visible"=w329) -> ()  [unwired: 2 in, 2 out]
        n201 = property on="Rev/Fwd" class="Clust (strict)"("Visible"=w329) -> ()  [unwired: 2 in, 2 out]
        n202 = property on="Ring" class="Ring (strict)"("Visible"=w329) -> ()  [unwired: 2 in, 2 out]
      }
      event "Listbox": Double Click {
        n203 = event-data() -> ("PlatMods.Shift"=w337:bool, "Row"=w339:i32)  [unwired: 1 in]
        n204 = case shown="False" w337 {
          tunnel: w339 -> [w343 _]
          tunnel: 1 -> [w342 _]
          frame False {
            n205 = property on="Listbox" class="LstBox (strict)"() -> ("Item Symbols"=w341:i32[])  [unwired: 2 in, 2 out]
            n206 = Replace Array Subset(array=w341, new element=w342, index=w343) -> (w340:i32[])
            n207 = property on="Listbox" class="LstBox (strict)"("Item Symbols"=w340) -> ()  [unwired: 2 in, 2 out]
          }
          frame True {
            w344 = 0 ("Top Row")
            n208 = property on="Listbox" class="LstBox (strict)"() -> ("Number of Rows"=w346:u32)  [unwired: 2 in, 2 out]
            n209 = Initialize Array(0, w346) -> (w345:i32[])
            n210 = property on="Listbox" class="LstBox (strict)"("Top Row"=w344, "Value"=w344, "Item Symbols"=w345) -> ()  [unwired: 2 in, 2 out]
          }
        }
      }
      event "Listbox": Key Down {
        n211 = event-data() -> ("VKey"=w350:T19)  [unwired: 1 in]
        n212 = case shown="\"Left\", \"Right\"" w350 {
          selector: w350 -> [w355 _]
          tunnel: eventvkey."Left" ("VKey") -> [w353 _]
          frame "Left", "Right" {
            n213 = Equal?(x=w353, y=w355) -> (x = y?=w354:bool)
            n214 = Select(t=0, s=w354, f=1) -> (s? t:f=w356:i32)
            n215 = property on="Listbox" class="LstBox (strict)"() -> ("Item Symbols"=w359:i32[])  [unwired: 2 in, 2 out]
            n216 = Replace Array Subset(array=w359, new element=w356, index="Listbox") -> (w358:i32[])
            n217 = property on="Listbox" class="LstBox (strict)"("Item Symbols"=w358) -> ()  [unwired: 2 in, 2 out]
          }
          frame Default {
          }
        }
      }
      event "DB Camera Config": Value Change {
        n218 = event-data() -> ("NewVal"=w363:bool)  [unwired: 1 in]
        n219 = case shown="False" w363 {
          tunnel: w362 -> [w372 _]
          tunnel: [w365 w383] -> w361
          tunnel: w360 -> [w364 w383]
          frame False {
            w379 = "Camera"
            w382 = FALSE ("Visible")
            n220 = local read "Camera Settings"() -> (w371:T1)
            n221 = Index Array(array=w372) -> (element=w375:cluster{string[]})  [unwired: 1 in]
            n222 = Unbundle(w371) -> ("Frate Rate"=w370:i32, "Compression"=w369:i32, "Size"=w373:u16)
            n223 = Unbundle(w375) -> (w374:string[])
            n224 = Index Array(array=w374, index=w373) -> (element=w368:string)
            n225 = call-poly <vilib>:"Write Key.vi"("section"=w379, "value"=w368, "key"="Size", "refnum"=w364) -> ("refnum out"=w381:T18)  [unwired: 2 in, 5 out]
            n226 = call-poly <vilib>:"Write Key.vi"("section"=w379, "value"=w370, "key"="FrameRate", "refnum"=w381) -> ("refnum out"=w380:T18)  [unwired: 1 in, 6 out]
            n227 = property on="Camera Settings" class="Clust (strict)"("Visible"=w382) -> ()  [unwired: 2 in, 2 out]
            n228 = local write "DB Camera Config"(w382) -> ()
            n229 = call-poly <vilib>:"Write Key.vi"("section"=w379, "value"=w369, "key"="Compression", "refnum"=w380) -> ("refnum out"=w366:T18)  [unwired: 1 in, 6 out]
            n230 = call <vilib>:"Close Config Data.vi"("refnum"=w366) -> ("file path"=w367:path)  [unwired: 2 in, 8 out]
            n231 = call <vilib>:"Open Config Data.vi"("configuration file path"=w367) -> ("refnum"=w365:T18)  [unwired: 8 in, 2 out]
          }
          frame True {
            n232 = property on="Camera Settings" class="Clust (strict)"("Visible"=TRUE) -> ()  [unwired: 2 in, 2 out]
          }
        }
      }
      event "Camera Settings": Value Change {
        n233 = event-data() -> ("NewVal"=w396:T1)  [unwired: 1 in]
        n234 = Index Array(array=w392) -> (element=w391:cluster{string[]})  [unwired: 1 in]
        n235 = Unbundle(w396) -> ("Frate Rate"=w387:i32, "Compression"=w386:i32, "Size"=w389:u16)
        n236 = Unbundle(w391) -> (w390:string[])
        n237 = Index Array(array=w390, index=w389) -> (element=w388:string)
        n238 = Format Into String(format string="%s   %dfps   %d%%", w388, w387, w386) -> (resulting string=w393:string)  [unwired: 2 in, 1 out]
        n239 = Build Array(w393) -> (w394:string[])
        n240 = property on="DB Camera Config" class="Bool (strict)"("Strings [4]"=w394) -> ()  [unwired: 2 in, 2 out]
      }
      event "Motor.Enable": Value Change {
        n241 = event-data() -> ("NewVal"=w402:bool)  [unwired: 1 in]
        n242 = Unbundle("Motor") -> ("Value"=w401:dbl)  [unwired: 1 out]
        n243 = Select(t=w401, s=w402, f=0.0) -> (s? t:f=w399:dbl)
        n244 = call <vilib>:"NT Write Number.vi"("Numeric"=w399, "Name"=w398) -> ()  [unwired: 9 in, 1 out]
      }
      event "Slider": Value Change {
        n245 = event-data() -> ("NewVal"=w405:dbl)  [unwired: 1 in]
        n246 = call <vilib>:"NT Write Number.vi"("Numeric"=w405, "Name"=w406) -> ()  [unwired: 9 in, 1 out]
      }
      event "On/Off": Value Change {
        n247 = event-data() -> ("NewVal"=w410:bool)  [unwired: 1 in]
        n248 = Boolean To (0,1)(Boolean=w410) -> (0, 1=w409:i16)
        n249 = call <vilib>:"NT Write Number.vi"("Numeric"=w409, "Name"=w408) -> ()  [unwired: 9 in, 1 out]
      }
      event "Rev/Fwd": Value Change {
        n250 = event-data() -> ("NewVal.Forward"=w418:bool, "NewVal.Reverse"=w417:bool)  [unwired: 1 in]
        n251 = Boolean To (0,1)(Boolean=w418) -> (0, 1=w414:i16)
        n252 = Boolean To (0,1)(Boolean=w417) -> (0, 1=w416:i16)
        n253 = Negate(x=w416) -> (-x=w415:i16)
        n254 = Add(x=w414, y=w415) -> (x+y=w413:i16)
        n255 = call <vilib>:"NT Write Number.vi"("Numeric"=w413, "Name"=w412) -> ()  [unwired: 9 in, 1 out]
      }
      event "Ring": Value Change {
        n256 = event-data() -> ("NewVal"=w422:u16)  [unwired: 1 in]
        n257 = property on="Ring" class="Ring (strict)"() -> ("Strings []"=w423:string[])  [unwired: 2 in, 2 out]
        n258 = Index Array(array=w423, index=w422) -> (element=w421:string)
        n259 = call <vilib>:"NT Write String.vi"("String"=w421, "Name"=w420) -> ()  [unwired: 9 in, 1 out]
      }
    }
  }
  n260 = Index Array(array=w13) -> (element=w14:cluster{string[]})  [unwired: 1 in]
  n261 = Unbundle(w14) -> (w12:string[])
  n262 = Match First String(2:w12, 3:w11) -> (0:w10:i32)  [unwired: 1 out]
  n263 = Bundle("value"=w16, "value"=w15, "index"=w10) -> (w4:cluster{"value":i32, "value":i32, "index":i32})  [unwired: 1 out]
  n264 = property on="On/Off" class="Bool (strict)"("Visible"=w27) -> ()  [unwired: 2 in, 2 out]
  n265 = property on="Motor" class="Clust (strict)"("Visible"=w27) -> ()  [unwired: 2 in, 2 out]
  n266 = property on="Progress" class="Clust (strict)"("Visible"=w27) -> ()  [unwired: 2 in, 2 out]
  n267 = property on="Ring" class="Ring (strict)"("Visible"=w27) -> ()  [unwired: 2 in, 2 out]
  n268 = property on="Camera Settings" class="Clust (strict)"("Val(Sgnl)"=w4) -> ()  [unwired: 2 in, 2 out]
  n269 = property on="Rev/Fwd" class="Clust (strict)"("Visible"=w27) -> ()  [unwired: 2 in, 2 out]
  n270 = property on="Camera Settings" class="Clust (strict)"("Visible"=w27) -> ()  [unwired: 2 in, 2 out]
  n271 = local write "DB Camera Config"(w27) -> ()
